vi "Blue RunLog Viewer Main.vi"() -> ()   [LabVIEW 2020, in "Blue RunLog Viewer.lvlib"]
uses:
  Blue RunLog Viewer.lvlib
  <userlib>/Blue Origin/RunLog_OpenSource/SubVIs/runlog logging levels.ctl
  <userlib>/Blue Origin/RunLog_OpenSource/SubVIs/runlog init options.ctl
  <userlib>/Blue Origin/RunLog_OpenSource/SubVIs/runlog decorate options.ctl
  <userlib>/Blue Origin/RunLog_OpenSource/Classes/RunLog/New.vi
  <userlib>/Blue Origin/RunLog_OpenSource/Classes/RunLog/Decorate.vi
  <userlib>/Blue Origin/RunLog_OpenSource/Classes/RunLog/Stop Load Stream.vi
  <userlib>/Blue Origin/RunLog_OpenSource/Classes/RunLog/Clear.vi
  <vilib>/Utility/libraryn.llb/Check if File or Folder Exists.vi
  <vilib>/Utility/file.llb/Is Path and Not Empty.vi
  <vilib>/Utility/libraryn.llb/Librarian Path Location.vi
  <userlib>/_OpenG.lib/file/file.llb/File Exists__ogtk.vi
  <userlib>/_OpenG.lib/file/file.llb/File Exists - Scalar__ogtk.vi
  <userlib>/Blue Origin/RunLog_OpenSource/Classes/RunLog/Load log.vi
  <userlib>/Blue Origin/RunLog_OpenSource/Classes/RunLog/Shutdown.vi
  <userlib>/Blue Origin/RunLog_OpenSource/Classes/RunLog/RunLog.lvclass
  <userlib>/Blue Origin/RunLog_OpenSource/RunLog.lvlib
panel:
  in  "Path":path
  in  "poll?":bool=TRUE caption="Poll?"
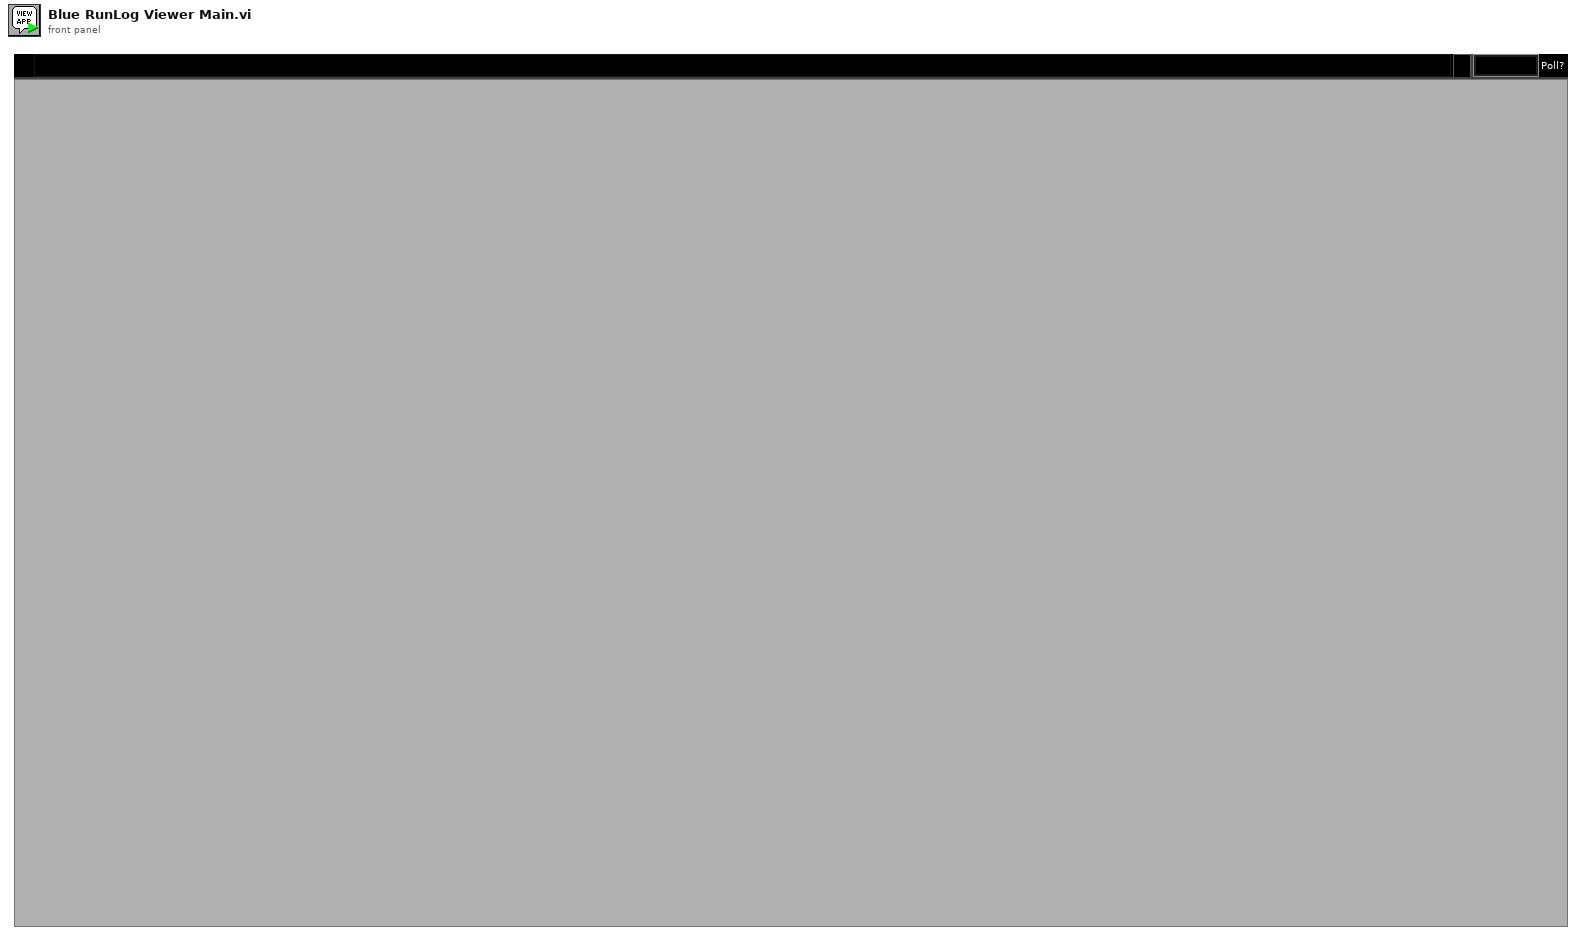
[diagram p1: front panel]
types:
  T1 = typedef "RunLog.lvlib/runlog decorate options.ctl" = enum16{"on (once)", "always off", "always on"}
  T2 = typedef "RunLog.lvlib/runlog logging levels.ctl" = enum16{"DEBUG", "INFO", "WARNING", "ERROR", "CRITICAL"}
  T3 = typedef "RunLog.lvlib/runlog init options.ctl" = cluster{"visible logging levels":T2[], "autoscroll?":bool, "UI visible? (T)":bool}
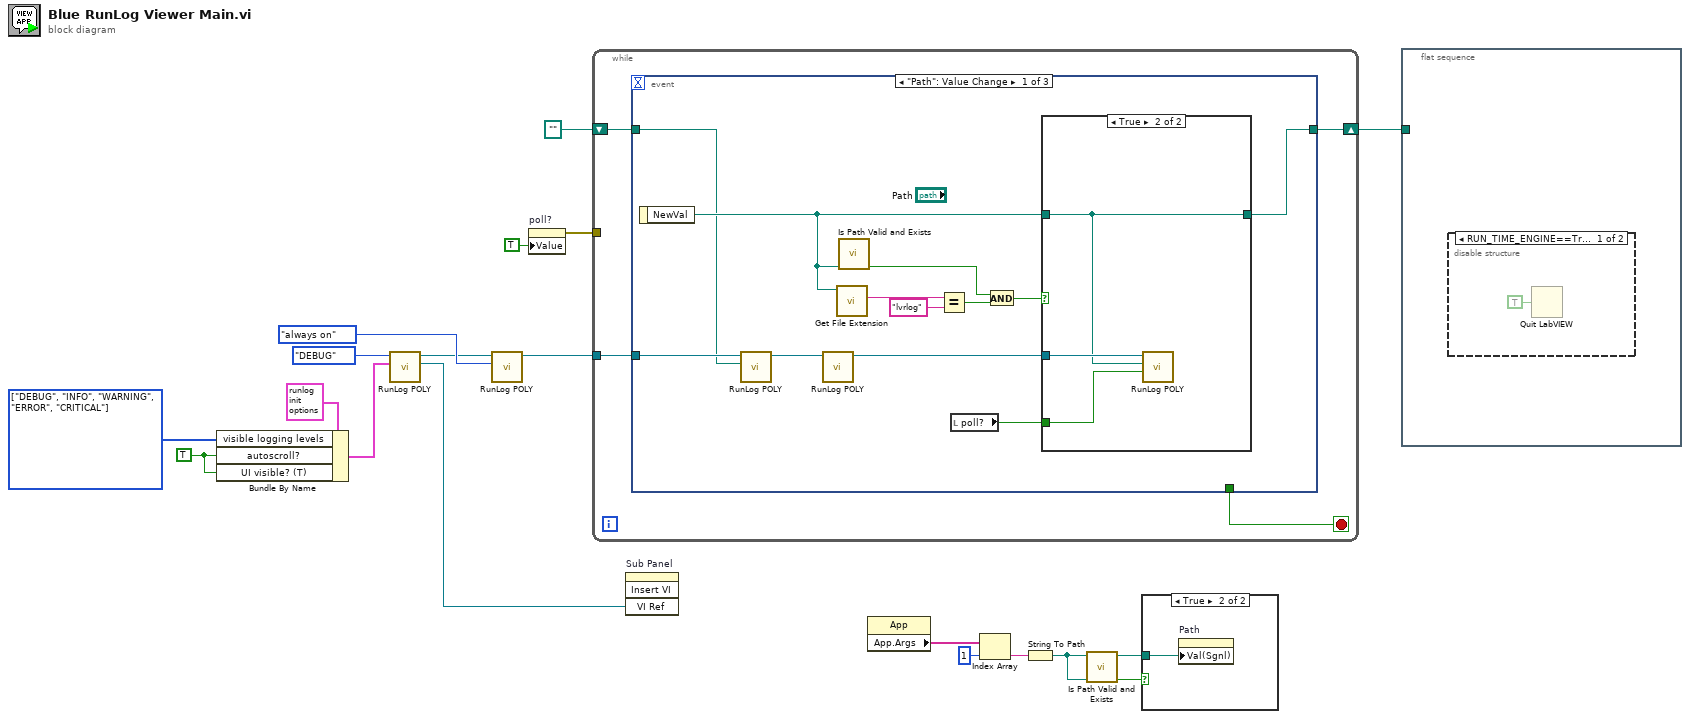
[diagram p0: block diagram]
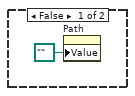
[diagram p3: hidden frame]
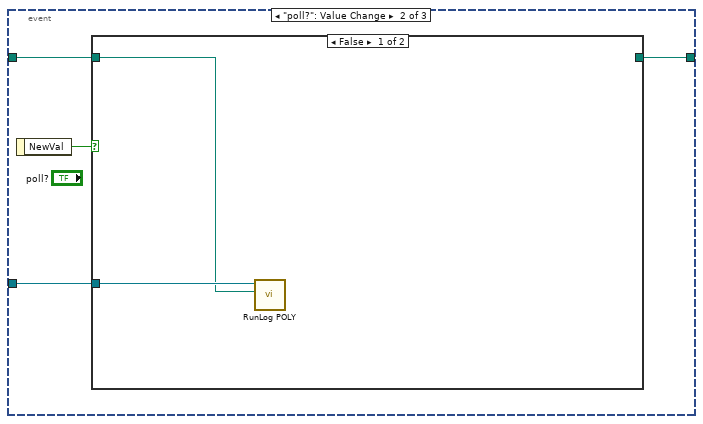
[diagram p5: hidden frame]
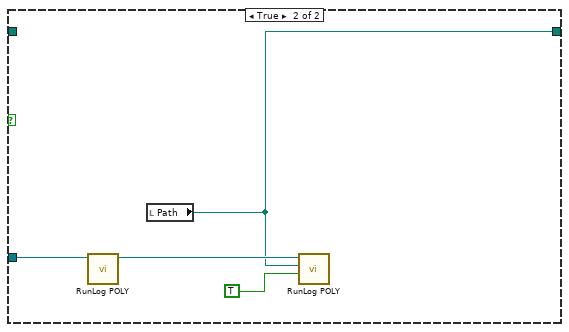
[diagram p6: hidden frame]
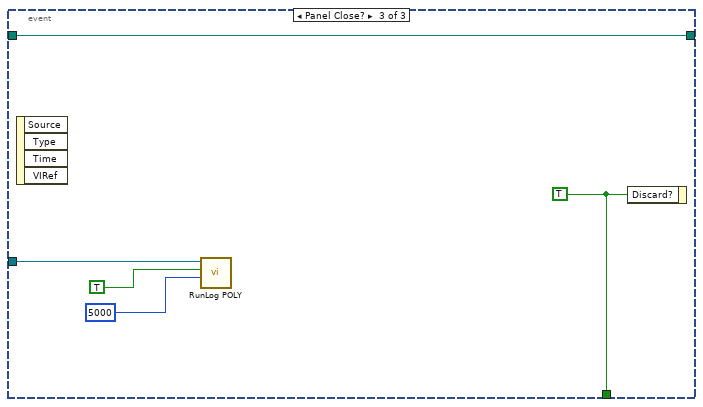
[diagram p7: hidden frame]
diagram:
  w5 = TRUE ("autoscroll?")
  w6 = T2[] [enum."DEBUG", enum."INFO", enum."WARNING", enum."ERROR", enum."CRITICAL"] items=["DEBUG", "INFO", "WARNING", "ERROR", "CRITICAL"] ("visible logging levels")
  n1 = Bundle By Name(cluster=T3 {"visible logging levels"=[enum."INFO", enum."WARNING", enum."ERROR", enum."CRITICAL"], "autoscroll?"=TRUE, "UI visible? (T)"=TRUE} ("Init options"), "visible logging levels"=w6, "autoscroll?"=w5, "UI visible? (T)"=w5) -> (w4:T3)
  n2 = call-poly <userlib>:"RunLog POLY.vi"("Init options"=w4, "Logging level"=runlog_logging_levels."DEBUG") -> ("VI Ref"=w9:refnum<vi>, "RunLog out"=w2:refnum<class "RunLog.lvclass">)  [unwired: 7 in, 1 out]
  n3 = call-poly <userlib>:"RunLog POLY.vi"("Action"=runlog_decorate_options."always on", "RunLog in"=w2) -> ("RunLog out"=w1:refnum<class "RunLog.lvclass">)  [unwired: 8 in, 1 out]
  n4 = property on="poll?" class="Bool (strict)"("Value"=TRUE ("poll?")) -> (error out=w11:errorcluster)  [unwired: 2 in, 1 out]
  n5 = while {
    tunnel: w1 -> [w22]
    shift-right: [w20] -> w10
    shift-left: path "" ("NewVal") -> [w21]
    tunnel: w11 -> [_]
    stop <- w19 stop-if-true
    n6 = event shown="[0] \"Path\": Value Change" {
      selector: _ -> [_ _ _]
      dyn-events: _ -> [_ _ _]
      timeout: _ -> [_ _ _]
      tunnel: w22 -> [w26 w41 w50]
      tunnel: w21 -> [w25 w39 w52]
      tunnel: [w27 w38 w52] -> w20
      tunnel: [_ _ w51] -> w19
      event "Path": Value Change {
        n7 = event-data() -> ("NewVal"=w29:path)  [unwired: 1 in]
        n8 = call-poly <userlib>:"RunLog POLY.vi"("log path (*.lvrelog)"=w25, "RunLog in"=w26) -> ("RunLog out"=w24:refnum<class "RunLog.lvclass">)  [unwired: 8 in, 1 out]
        n9 = call-poly <userlib>:"RunLog POLY.vi"("RunLog in"=w24) -> ("RunLog out"=w23:refnum<class "RunLog.lvclass">)  [unwired: 9 in, 1 out]
        n10 = call <vilib>:"Get File Extension.vi"("file"=w29) -> ("lowercase file extension"=w34:string)  [unwired: 6 in, 4 out]
        n11 = call <userlib>:"Is Path Valid and Exists.vi"("File/Folder Path"=w29) -> ("Valid and Exists?"=w31:bool)  [unwired: 9 in, 1 out]
        n12 = Equal?(x=w34, y="lvrlog") -> (x = y?=w32:bool)
        n13 = local read "poll?"() -> (w28:bool)
        n14 = And(x=w31, y=w32) -> (x .and. y?=w30:bool)
        n15 = case shown="True" w30 {
          tunnel: w23 -> [_ w37]
          tunnel: w29 -> [_ w36]
          tunnel: w28 -> [_ w35]
          tunnel: [_ w36] -> w27
          frame False {
          }
          frame True {
            n16 = call-poly <userlib>:"RunLog POLY.vi"("Stream loading? (F)"=w35, "log path (*.lvrelog)"=w36, "RunLog in"=w37) -> ()  [unwired: 7 in, 2 out]
          }
        }
      }
      event "poll?": Value Change {
        n17 = event-data() -> ("NewVal"=w40:bool)  [unwired: 1 in]
        n18 = case shown="False" w40 {
          tunnel: w41 -> [w43 w47]
          tunnel: w39 -> [w42 _]
          tunnel: [_ w45] -> w38
          frame False {
            n19 = call-poly <userlib>:"RunLog POLY.vi"("log path (*.lvrelog)"=w42, "RunLog in"=w43) -> ()  [unwired: 8 in, 2 out]
          }
          frame True {
            n20 = call-poly <userlib>:"RunLog POLY.vi"("RunLog in"=w47) -> ("RunLog out"=w46:refnum<class "RunLog.lvclass">)  [unwired: 9 in, 1 out]
            n21 = local read "Path"() -> (w45:path)
            n22 = call-poly <userlib>:"RunLog POLY.vi"("Stream loading? (F)"=TRUE, "log path (*.lvrelog)"=w45, "RunLog in"=w46) -> ()  [unwired: 7 in, 2 out]
          }
        }
      }
      event Panel Close? {
        w51 = TRUE ("Discard?")
        n23 = event-data() -> ()  [unwired: 1 in, 4 out]
        n24 = call-poly <userlib>:"RunLog POLY.vi"("timeout in ms (-1)"=5000 ("wait timeout in ms (-1)"), "Wait until finished?"=TRUE ("Wait until shutdown? (F)"), "RunLog in"=w50) -> ()  [unwired: 6 in, 3 out]
        n25 = event-data("Discard?"=w51) -> ()  [unwired: 1 in, 1 out]
      }
    }
  }
  n26 = invoke on="Sub Panel" class="SubPnl" method="Insert VI"("VI Ref"=w9) -> ()  [unwired: 3 in, 4 out]
  n27 = property class="App"() -> ("App.Args"=w17:string[])  [unwired: 2 in, 2 out]
  n28 = Index Array(array=w17, index=1) -> (element=w16:string)
  n29 = String To Path(string=w16) -> (path=w14:path)
  n30 = call <userlib>:"Is Path Valid and Exists.vi"("File/Folder Path"=w14) -> ("Valid and Exists?"=w15:bool)  [unwired: 9 in, 1 out]
  n31 = case shown="True" w15 {
    tunnel: w14 -> [_ w54]
    frame False {
      n32 = property on="Path" class="Path"("Value"=path "" ("Path")) -> ()  [unwired: 2 in, 2 out]
    }
    frame True {
      n33 = property on="Path" class="Path"("Val(Sgnl)"=w54) -> ()  [unwired: 2 in, 2 out]
    }
  }
  n34 = flat-sequence {
    tunnel: w10 -> [_]
    frame #0 {
      n35 = disable-structure shown="RUN_TIME_ENGINE==True, Default" {
        frame condition #0 {
          n36 = Quit LabVIEW(quit? (T)=TRUE) -> ()
        }
        frame condition #1 (active) {
        }
      }
    }
  }
